vi "Average_Error.vi"(11 "WaveformChart in":refnum<vi>) -> (1 "Std deviation diff":dbl format="%0.2f", 2 "Std measured (px)":dbl format="%0.2f", 3 "Avg Error (px)":dbl format="%0.2f")   [LabVIEW 2020]
uses:
  <vilib>/Analysis/NI_AALBase.lvlib
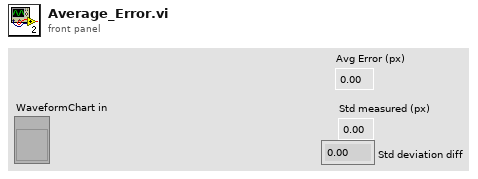
[diagram p1: front panel]
types:
  T1 = cluster{"X Centroid":dbl, "X Centroid":dbl, "X Centroid":sgl, "Y Centroid":sgl}[]
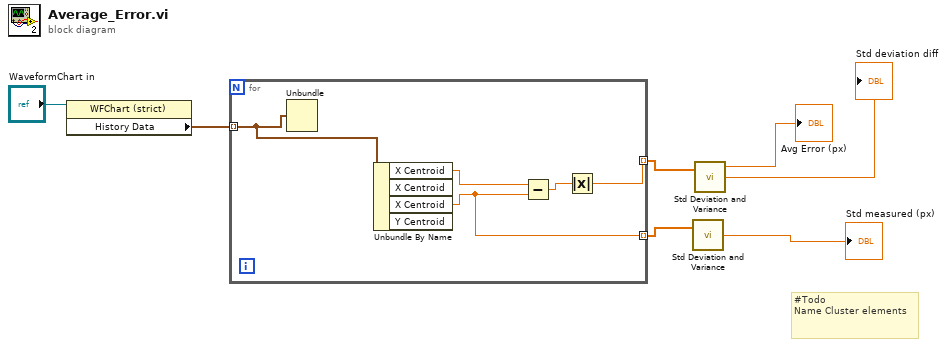
[diagram p0: block diagram]
diagram:
  # "#Todo\nName Cluster elements"
  n1 = property on="Property Node" class="WFChart (strict)"(reference="WaveformChart in") -> ("History Data"=w6:T1)  [unwired: 1 in, 2 out]
  n2 = for {
    tunnel: w6 -> [w12] mode=indexing
    tunnel: [w9] -> w5 mode=indexing
    tunnel: [w8] -> w3 mode=indexing
    n3 = Unbundle(w12) -> ()  [unwired: 4 out]
    n4 = Unbundle By Name(w12) -> ("X Centroid"=w11:dbl, "X Centroid"=w8:sgl)  [unwired: 2 out]
    n5 = Subtract(x=w11, y=w8) -> (x-y=w10:dbl)
    n6 = Absolute Value(x=w10) -> (abs(x)=w9:dbl)
  }
  n7 = call <vilib>:"Std Deviation and Variance.vi"("X"=w3) -> ("standard deviation"=→"Std measured (px)":dbl)  [unwired: 1 in, 2 out]
  n8 = call <vilib>:"Std Deviation and Variance.vi"("X"=w5) -> ("mean"=→"Avg Error (px)":dbl, "standard deviation"=→"Std deviation diff":dbl)  [unwired: 1 in, 1 out]
